vi "Rename Library.vi"(0 "generation data":T1, 3 "error in":errorcluster) -> (7 "generation data out":T1, 10 "error out":errorcluster)   [LabVIEW 2024, in "gRPC Client Generation.lvlib"]
uses:
  gRPC Client Generation.lvlib
  Generation Data.ctl
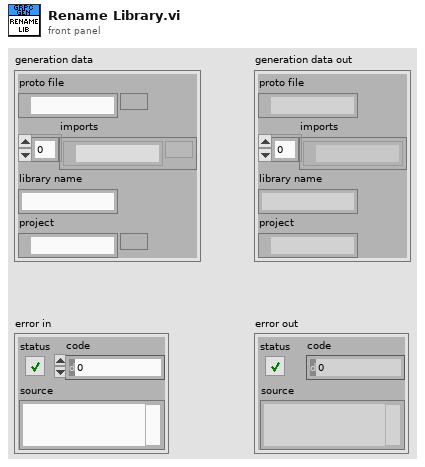
[diagram p1: front panel]
types:
  T1 = typedef "gRPC Client Generation.lvlib/Generation Data.ctl" = cluster{"proto file":path, "imports":path[], "library name":string, "project":path}
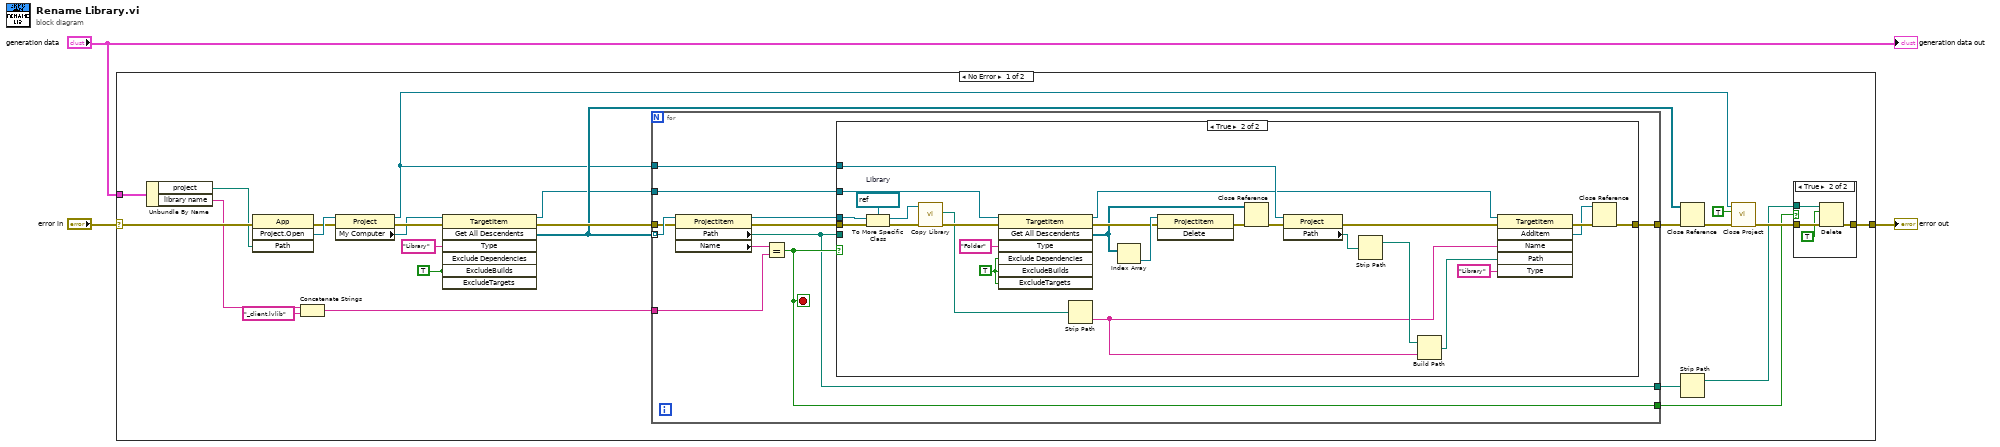
[diagram p0: block diagram]
diagram:
  n1 = case shown="No Error" "error in" {
    selector: "error in" -> [w26 w71]
    tunnel: "generation data" -> [w27 _]
    tunnel: [w25 w71] -> w2
    frame No Error {
      w15 = TRUE ("ExcludeDependencies")
      n2 = Unbundle By Name(w27) -> ("project"=w18:path, "library name"=w14:string)
      n3 = invoke class="App" method="Project.Open"(error in=w26, "Path"=w18) -> (error out=w17:errorcluster, "Project:Open"=w24:refnum<vi>)  [unwired: 2 in, 2 out]
      n4 = Concatenate Strings(w14, "_client.lvlib" ("format string")) -> (w19:string)
      n5 = property class="Project"(reference=w24, error in=w17) -> (reference out=w8:refnum<vi>, error out=w23:errorcluster, "My Computer"=w22:refnum<vi>)
      n6 = invoke class="TargetItem" method="Get All Descendents"(reference=w22, error in=w23, "Type"="Library", "Exclude Dependencies"=w15, "ExcludeBuilds"=w15, "ExcludeTargets"=w15) -> (reference out=w9:refnum<vi>, error out=w16:errorcluster, "All Descendents"=w12:refnum<vi>[])  [unwired: 1 in, 4 out]
      n7 = for {
        tunnel: w12 -> [w43] mode=indexing
        tunnel: w19 -> [w42]
        tunnel: w16 -> [w41]
        tunnel: [w39] -> w13
        tunnel: [w38] -> w7
        tunnel: [w37] -> w6
        tunnel: w9 -> [w34]
        tunnel: w8 -> [w33]
        stop <- w38 stop-if-true
        n8 = property class="ProjectItem"(reference=w43, error in=w41) -> (reference out=w35:refnum<vi>, error out=w36:errorcluster, "Path"=w37:path, "Name"=w40:string)
        n9 = Equal?(x=w40, y=w42) -> (x = y?=w38:bool)
        n10 = case shown="True" w38 {
          tunnel: w36 -> [w44 w70]
          tunnel: w37 -> [_ _]
          tunnel: [w44 w46] -> w39
          tunnel: w35 -> [_ w68]
          tunnel: w34 -> [_ w67]
          tunnel: w33 -> [_ w66]
          frame False {
          }
          frame True {
            w60 = TRUE ("ExcludeBuilds")
            w65 = refnum<vi> refnum  # Library
            n11 = To More Specific Class(target class=w65, reference=w68, error in=w70) -> (specific class reference=w64:refnum<vi>, error out=w63:errorcluster)
            n12 = call "Copy Library.vi"("error in"=w63, "library"=w64) -> ("error out"=w62:errorcluster, "New Library Path"=w52:path)  [unwired: 7 in, 1 out]
            n13 = invoke class="TargetItem" method="Get All Descendents"(reference=w67, error in=w62, "Type"="Folder", "Exclude Dependencies"=w60, "ExcludeBuilds"=w60, "ExcludeTargets"=w60) -> (reference out=w55:refnum<vi>, error out=w58:errorcluster, "All Descendents"=w56:refnum<vi>[])  [unwired: 1 in, 4 out]
            n14 = Strip Path(path=w52) -> (name=w49:string)  [unwired: 1 out]
            n15 = Index Array(array=w56) -> (element=w59:refnum<vi>)  [unwired: 1 in]
            n16 = invoke class="ProjectItem" method="Delete"(reference=w59, error in=w58) -> (error out=w57:errorcluster)  [unwired: 1 in, 2 out]
            n17 = Close Reference(reference=w56, error in (no error)=w57) -> (error out=w48:errorcluster)
            n18 = property class="Project"(reference=w66, error in=w48) -> (error out=w47:errorcluster, "Path"=w53:path)  [unwired: 1 out]
            n19 = Strip Path(path=w53) -> (stripped path=w51:path)  [unwired: 1 out]
            n20 = Build Path(base path=w51, name or relative path=w49) -> (appended path=w50:path)
            n21 = invoke class="TargetItem" method="AddItem"(reference=w55, error in=w47, "Name"=w49, "Path"=w50, "Type"="Library") -> (error out=w69:errorcluster, "AddItem"=w45:refnum<vi>)  [unwired: 1 in, 4 out]
            n22 = Close Reference(reference=w45, error in (no error)=w69) -> (error out=w46:errorcluster)
          }
        }
      }
      n23 = Close Reference(reference=w12, error in (no error)=w13) -> (error out=w11:errorcluster)
      n24 = Strip Path(path=w6) -> (stripped path=w5:path)  [unwired: 1 out]
      n25 = call "Close Project.vi"("error in"=w11, "save"=TRUE, "project ref"=w8) -> ("error out"=w10:errorcluster)  [unwired: 8 in]
      n26 = case shown="True" w7 {
        tunnel: w10 -> [w28 w32]
        tunnel: [w28 w31] -> w25
        tunnel: w5 -> [_ w29]
        frame False {
        }
        frame True {
          n27 = Delete(path (use dialog)=w29, entire hierarchy (F)=TRUE, error in=w32) -> (error out=w31:errorcluster)  [unwired: 2 in, 2 out]
        }
      }
    }
    frame Error {
    }
  }
  "error out" <- w2
  "generation data out" <- "generation data"
